vi "Channel Selection Dialog.vi"(7 "DisplayFilter":u8(ring)=7 items=["K_CHAN_R", "K_CHAN_W", "K_CHAN_RW", "K_CHAN_VOLT", "K_CHAN_FAULT", "K_ALL", "K_CUSTOM", "K_CHAN_R_VIS", "K_CHAN_W_VIS", "K_CHAN_RW_VIS", "K_CHAN_VOLT_VIS", "K_CHAN_FAULT_VIS"], 8 "error in (no error)":errorcluster, 10 "Current selection":string, 11 "NIVS.System Definition Root":refnum<k24>) -> (0 "error out":errorcluster, 1 "Cancelled":bool, 2 "New selection":string)   [LabVIEW 2012]
doc: "Use this template to create a dialog box with event handling."
uses:
  NationalInstruments.VeriStand.SystemStorageUI
  NationalInstruments.VeriStand.SystemStorage
  NationalInstruments.VeriStand
  <vilib>/NI Veristand/UI Controls/Single Node Browser/NI_VS UI Single Node Browser.lvlib
panel:
  in  "Cancel":bool
  in  "Ok":bool
  in  "Selected Channel":refnum<k24>(container)
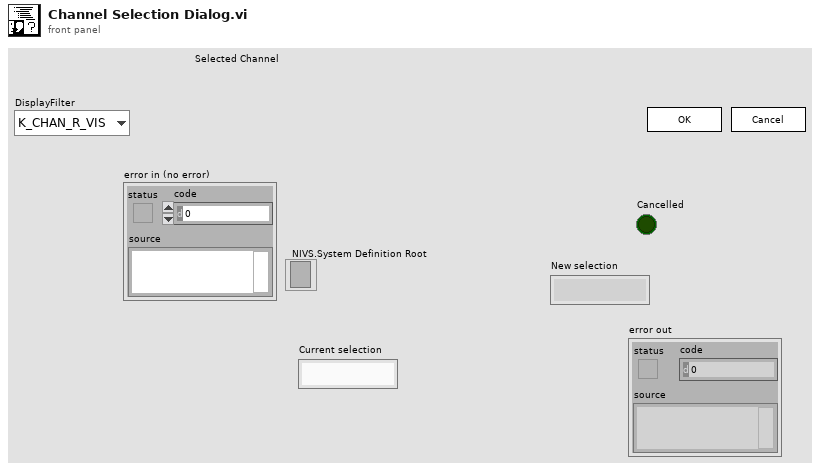
[diagram p1: front panel]
types:
  T1 = typedef "NI_VS UI Single Node Browser.lvlib/Callback Type.ctl" = cluster{"Net Callbacks":refnum<k27>[], "Event":refnum<user-event>}
  T2 = typedef "NI_VS UI Single Node Browser.lvlib/Node Ref.ctl" = refnum<k24>
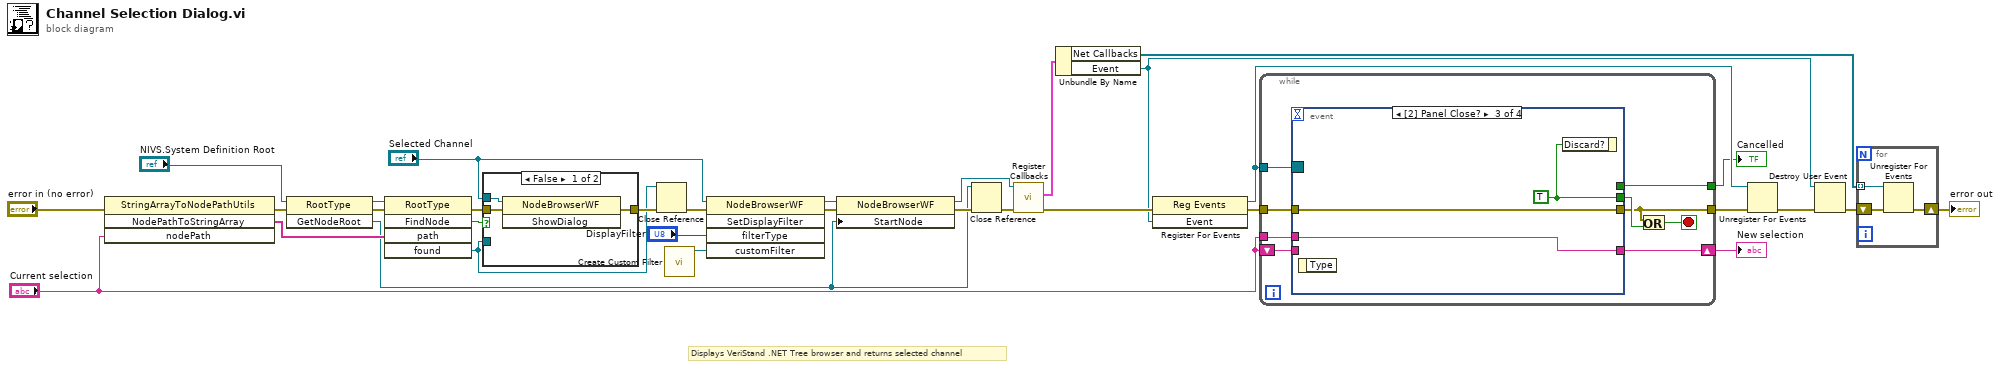
[diagram p0: block diagram]
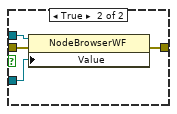
[diagram p2: hidden frame]
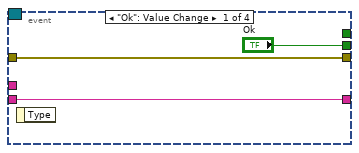
[diagram p3: hidden frame]
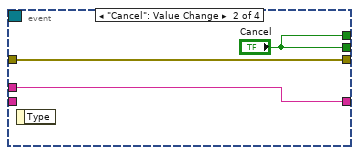
[diagram p4: hidden frame]
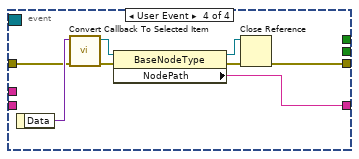
[diagram p5: hidden frame]
diagram:
  # "Displays VeriStand .NET Tree browser and returns selected channel"
  n1 = invoke class="StringArrayToNodePathUtils" method="NodePathToStringArray"(error in="error in (no error)", "nodePath"="Current selection") -> (error out=w13:errorcluster, "NodePathToStringArray"=w12:string[])  [unwired: 2 in, 2 out]
  n2 = invoke class="RootType" method="GetNodeRoot"(reference="NIVS.System Definition Root", error in=w13) -> (reference out=w31:refnum<k24>, error out=w32:errorcluster, "GetNodeRoot"=w8:refnum<k24>)  [unwired: 1 in]
  n3 = invoke class="RootType" method="FindNode"(reference=w31, error in=w32, "path"=w12) -> (error out=w27:errorcluster, "FindNode"=w26:bool, "found"=w10:refnum<k24>)  [unwired: 2 in, 2 out]
  n4 = case shown="False" w26 {
    tunnel: w10 -> [_ w38]
    tunnel: w27 -> [w36 w39]
    tunnel: [w34 w37] -> w23
    tunnel: "Selected Channel" -> [w35 w40]
    frame False {
      n5 = invoke class="NodeBrowserWF" method="ShowDialog"(reference=w35, error in=w36) -> (error out=w34:errorcluster)  [unwired: 1 in, 2 out]
    }
    frame True {
      n6 = property class="NodeBrowserWF"(reference=w40, error in=w39, "Value"=w38) -> (error out=w37:errorcluster)  [unwired: 1 out]
    }
  }
  n7 = Close Reference(reference=w10, error in (no error)=w23) -> (error out=w3:errorcluster)
  n8 = call "Create Custom Filter.vi"() -> ("Custom Channel Alias Filter"=w2:refnum<k24>)  [unwired: 10 in, 1 out]
  n9 = invoke class="NodeBrowserWF" method="SetDisplayFilter"(reference="Selected Channel", error in=w3, "filterType"="DisplayFilter", "customFilter"=w2) -> (reference out=w6:refnum<k24>, error out=w5:errorcluster)  [unwired: 1 in, 3 out]
  n10 = property class="NodeBrowserWF"(reference=w6, error in=w5, "StartNode"=w8) -> (reference out=w28:refnum<k24>, error out=w29:errorcluster)
  n11 = Close Reference(reference=w8, error in (no error)=w29) -> (error out=w9:errorcluster)
  n12 = call <vilib>:"Register Callbacks.vi"("error in (no error)"=w9, "Single Node Browser"=w28) -> ("error out"=w33:errorcluster, "Callbacks"=w30:T1)  [unwired: 7 in, 1 out]
  n13 = Unbundle By Name(w30) -> ("Net Callbacks"=w18:refnum<k27>[], "Event"=w17:refnum<user-event>)
  n14 = register-events(error in=w33, w17) -> (reference out=w20:refnum<event-registration>, error out=w24:errorcluster)  [unwired: 1 in]
  n15 = while {
    tunnel: [w42] -> w22
    tunnel: w24 -> [w48]
    tunnel: w20 -> [w46]
    shift-right: [w45] -> w25
    shift-left: "Current selection" -> [w44]
    tunnel: "Current selection" -> [w43]
    tunnel: [w41] -> w7
    stop <- w47 stop-if-true
    n16 = event shown="[2] Panel Close?" {
      selector: w46 -> [_ _ _ _]
      dyn-events: _ -> [_ _ _ _]
      timeout: _ -> [_ _ _ _]
      tunnel: ["Ok" "Cancel" w58 _] -> w49
      tunnel: [w52 w55 w57 w64] -> w42
      tunnel: w48 -> [w52 w55 w57 w65]
      tunnel: [w50 w54 w56 w59] -> w45
      tunnel: w44 -> [w50 _ _ _]
      tunnel: w43 -> [_ w54 w56 _]
      tunnel: [_ "Cancel" _ _] -> w41
      event "Ok": Value Change {
        n17 = event-data() -> ()  [unwired: 1 in, 1 out]
      }
      event "Cancel": Value Change {
        n18 = event-data() -> ()  [unwired: 1 in, 1 out]
      }
      event Panel Close? {
        w58 = TRUE ("Cancel")
        n19 = event-data() -> ()  [unwired: 1 in, 1 out]
        n20 = event-data("Discard?"=w58) -> ()  [unwired: 1 in, 1 out]
      }
      event User Event {
        n21 = event-data() -> ("Data"=w66:variant)  [unwired: 1 in]
        n22 = call <vilib>:"Convert Callback To Selected Item.vi"("error in"=w65, "Data"=w66) -> ("error out"=w60:errorcluster, "Selected Item"=w63:T2)  [unwired: 8 in]
        n23 = property class="BaseNodeType"(reference=w63, error in=w60) -> (reference out=w62:T2, error out=w61:errorcluster, "NodePath"=w59:string)
        n24 = Close Reference(reference=w62, error in (no error)=w61) -> (error out=w64:errorcluster)
      }
    }
    n25 = Or(x=w42, y=w49) -> (x .or. y?=w47:bool)
  }
  "New selection" <- w25
  "Cancelled" <- w7
  n26 = Unregister For Events(event registration refnum=w20, error in=w22) -> (error out=w21:errorcluster)
  n27 = Destroy User Event(user event=w17, error in=w21) -> (error out=w19:errorcluster)
  n28 = for {
    tunnel: w18 -> [w68] mode=indexing
    shift-right: [w67] -> w11
    shift-left: w19 -> [w69]
    n29 = Unregister For Events(event registration refnum=w68, error in=w69) -> (error out=w67:errorcluster)
  }
  "error out" <- w11
